vi "check_API_Key.vi"(1 "API-key":string) -> (0 "Is_wrong_Key":bool)   [LabVIEW 2024]
uses:
  <vilib>/httpClient/LabVIEWHTTPClient.lvlib
panel:
  out "body":string
  out "headers":string
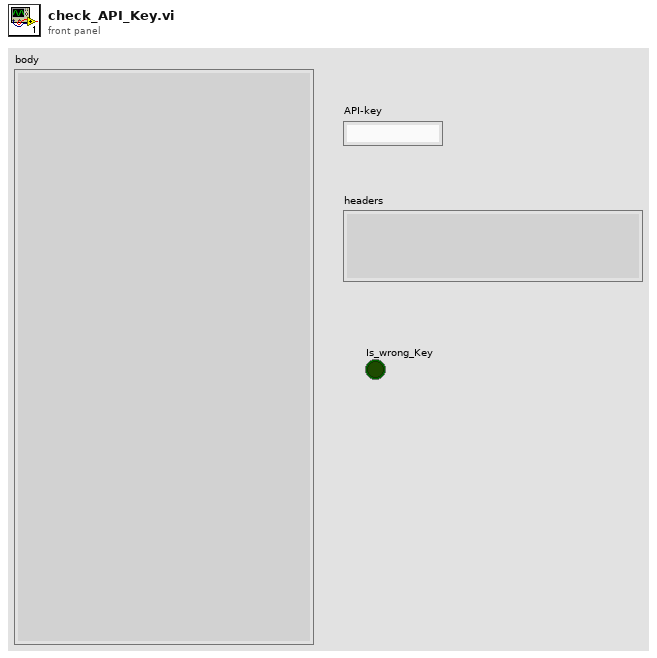
[diagram p1: front panel]
types:
  T1 = typedef "LabVIEWHTTPClient.lvlib/ClientHandle.ctl" = refnum<k1>
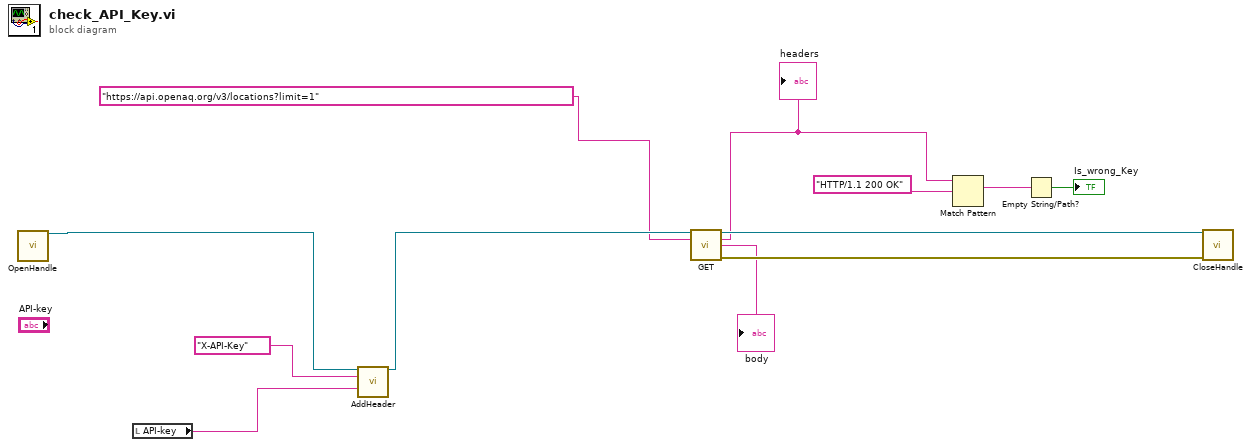
[diagram p0: block diagram]
diagram:
  n1 = call <vilib>:"OpenHandle.vi"() -> ("client handle out"=w10:T1)  [unwired: 14 in, 1 out]
  n2 = local read "API-key"() -> (w7:string)
  n3 = call <vilib>:"AddHeader.vi"("client handle"=w10, "header"="X-API-Key", "value"=w7) -> ("client handle out"=w8:T1)  [unwired: 11 in, 1 out]
  n4 = call <vilib>:"GET.vi"("client handle"=w8, "url"="https://api.openaq.org/v3/locations?limit=1") -> ("client handle out"=w12:T1, "headers"=w4:string, "body"=→"body":string, "error out"=w11:errorcluster)  [unwired: 10 in]
  "headers" <- w4
  n5 = Match Pattern(string=w4, regular expression="HTTP/1.1 200 OK") -> (match substring=w2:string)  [unwired: 1 in, 3 out]
  n6 = Empty String/Path?(string/path=w2) -> (empty?=→"Is_wrong_Key":bool)
  n7 = call <vilib>:"CloseHandle.vi"("client handle"=w12, "error in (no error)"=w11) -> ()  [unwired: 13 in, 1 out]
